vi "Stage.Settings.vi"(7 "Action":enum8{"Get", "Set"}(ring), 8 "error in (no error)":errorcluster, 10 "Settings":T1, 11 "Item Ref in":T4 format="%.0x") -> (0 "error out":errorcluster, 2 "Settings":T1, 3 "Item Ref out":T4 format="%.0x")   [LabVIEW 2015, in "Fuel Injection Addon System Explorer.lvlib"]
uses:
  Fuel Injection Addon System Explorer.lvlib
  <vilib>/NI Veristand/Custom Device API/Custom Device Item Ref.ctl
  Types/Stage.Settings.ctl
  Shared/Types/Stage.PullIn.Types.ctl
  Shared/Types/Stage.Transition.Types.ctl
  Shared/Constants.vi
  <vilib>/NI Veristand/Custom Device API/Get Item Property (U32).vi
  <vilib>/NI Veristand/Custom Device API/Set Item Property (U32).vi
  <vilib>/NI VeriStand/Custom Device API/Custom Device API.lvlib
  Shared/Fuel Injection Addon Shared.lvlib
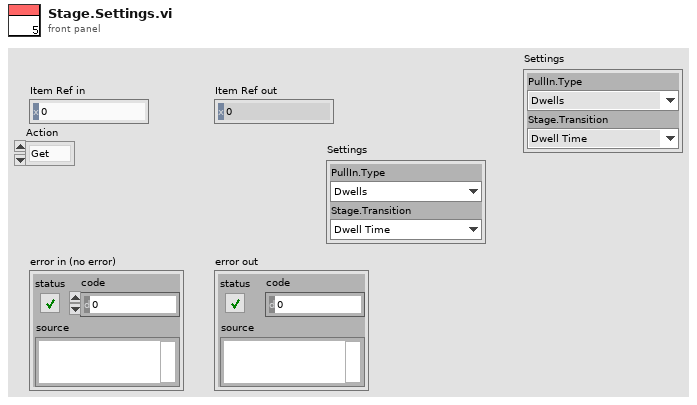
[diagram p1: front panel]
types:
  T1 = typedef "Fuel Injection Addon System Explorer.lvlib/Stage.Settings.ctl" = cluster{"PullIn.Type":T2, "Stage.Transition":T3}
  T2 = typedef "Stage.PullIn.Types.ctl" = enum8{"Dwells", "Current Drop"}
  T3 = typedef "Stage.Transition.Types.ctl" = enum8{"Dwell Time", "Voltage Level"}
  T4 = typedef "Custom Device API.lvlib/Custom Device Item Ref.ctl" = u64
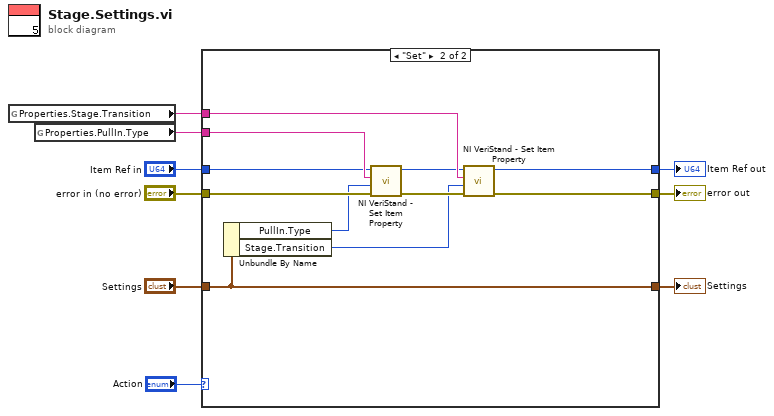
[diagram p0: block diagram]
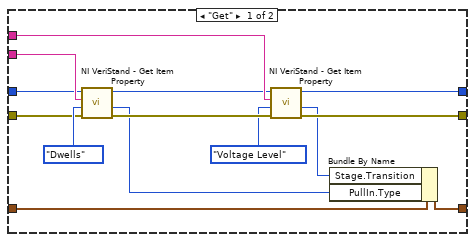
[diagram p2: hidden frame]
diagram:
  n1 = global read "Constants.vi" "Properties.Stage.Transition"() -> (w9:string)
  n2 = global read "Constants.vi" "Properties.PullIn.Type"() -> (w8:string)
  n3 = case shown="\"Set\"" "Action" {
    tunnel: w9 -> [w22 w33]
    tunnel: w8 -> [w21 w32]
    tunnel: [w20 w31] -> w7
    tunnel: [w18 w29] -> w6
    tunnel: "Item Ref in" -> [w16 w28]
    tunnel: "error in (no error)" -> [w14 w27]
    tunnel: "Settings" -> [w13 w24]
    tunnel: [w10 w24] -> w2
    frame "Get" {
      n4 = call-poly <vilib>:"NI VeriStand - Get Item Property.vi"("error in (no error)"=w14, "Default Value"=Stage.PullIn.Types."Dwells" ("PullIn.Type"), "Property Name"=w21, "Item Ref in"=w16) -> ("error out"=w23:errorcluster, "Value"=w12:u32, "Item Ref out"=w19:T4)  [unwired: 4 in, 1 out]
      n5 = call-poly <vilib>:"NI VeriStand - Get Item Property.vi"("error in (no error)"=w23, "Default Value"=Stage.Transition.Types."Voltage Level" ("Stage.Transition"), "Property Name"=w22, "Item Ref in"=w19) -> ("error out"=w18:errorcluster, "Value"=w11:u32, "Item Ref out"=w20:T4)  [unwired: 4 in, 1 out]
      n6 = Bundle By Name(cluster=w13, "Stage.Transition"=w11, "PullIn.Type"=w12) -> (w10:T1)
    }
    frame "Set" {
      n7 = Unbundle By Name(w24) -> ("PullIn.Type"=w25:T2, "Stage.Transition"=w26:T3)
      n8 = call-poly <vilib>:"NI VeriStand - Set Item Property.vi"("error in (no error)"=w27, "Value"=w25, "Property Name"=w32, "Item Ref in"=w28) -> ("error out"=w34:errorcluster, "Item Ref out"=w30:T4)  [unwired: 5 in, 1 out]
      n9 = call-poly <vilib>:"NI VeriStand - Set Item Property.vi"("error in (no error)"=w34, "Value"=w26, "Property Name"=w33, "Item Ref in"=w30) -> ("error out"=w29:errorcluster, "Item Ref out"=w31:T4)  [unwired: 5 in, 1 out]
    }
  }
  "Item Ref out" <- w7
  "error out" <- w6
  "Settings" <- w2
